vi "Write Numeric Range to Source (Base08 I16).vi"(4 "min":i16 format="%d bytes", 5 "<= max? (F)":bool, 6 "max":i16 format="%d bytes", 7 ">= min? (F)":bool, 8 "width (-)":i16, 9 "offset":i32, 10 "value":i16 format="%d bytes", 11 "error in":errorcluster) -> (1 "new offset":i32, 3 "error out":errorcluster)   [LabVIEW 2020, in "Static Errors.lvlib"]
doc: "Writes a string in the form of <b>min</b> <=/< <b>value</b> <=/< <b>max</b> to the source string of the provided <b>error cluster</b> at the specified <b>offset</b>."
uses:
  Static Errors.lvlib
  Write Numeric Scalar to Source (Base08 I16).vi
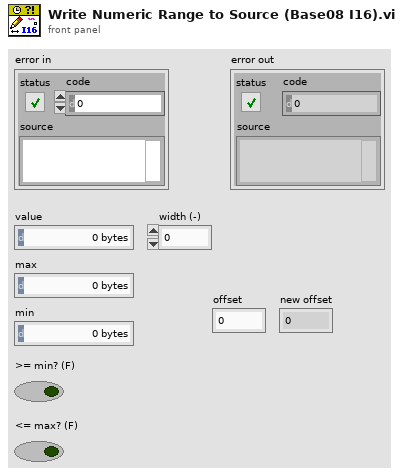
[diagram p1: front panel]
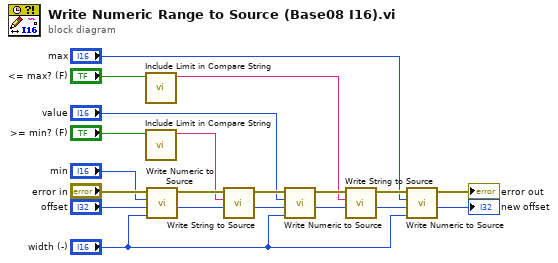
[diagram p0: block diagram]
diagram:
  n1 = call "Include Limit in Compare String.vi"("include limit in compare"="<= max? (F)") -> ("compare"=w1:string)  [unwired: 10 in]
  n2 = call "Include Limit in Compare String.vi"("include limit in compare"=">= min? (F)") -> ("compare"=w2:string)  [unwired: 10 in]
  n3 = call-poly "Write Numeric to Source.vi"("width (-)"="width (-)", "offset"="offset", "value"="min", "error in"="error in") -> ("new offset"=w19:i32, "error out"=w20:errorcluster)  [unwired: 6 in]
  n4 = call "Write String to Source.vi"("offset"=w19, "string"=w2, "error in"=w20) -> ("new offset"=w17:i32, "error out"=w18:errorcluster)  [unwired: 7 in]
  n5 = call-poly "Write Numeric to Source.vi"("width (-)"="width (-)", "offset"=w17, "value"="value", "error in"=w18) -> ("new offset"=w15:i32, "error out"=w16:errorcluster)  [unwired: 6 in]
  n6 = call "Write String to Source.vi"("offset"=w15, "string"=w1, "error in"=w16) -> ("new offset"=w13:i32, "error out"=w14:errorcluster)  [unwired: 7 in]
  n7 = call-poly "Write Numeric to Source.vi"("width (-)"="width (-)", "offset"=w13, "value"="max", "error in"=w14) -> ("new offset"=→"new offset":i32, "error out"=→"error out":errorcluster)  [unwired: 6 in]
